vi "斯坦道XML解析.vi"(10 "添加的路径":path, 11 "参数簇":T1={"启动模式"=enum."跨度核查", "启动参数"=1, "量程"=enum."低量程"} {"启动参数" items=["总磷"=1, "总氮"=2, "氨氮"=3]}) -> (2 "步骤时间":string[](array[string]), 3 "步骤名":string[](array[string]))   [LabVIEW 2016, in "斯坦道总氮.lvlib"]
uses:
  <vilib>/xml/Load XML File.vi
  <vilib>/xml/Close Reference(Node).vi
  <resource>/objmgr/DOMUserDefRef.rc
  <vilib>/xml/NI_XML.lvlib
panel:
  out "连接的字符串":string
  out "大小":i32
  out "XML字符串":string="<?xml version=\"1.0\" encoding=\"ISO-8859-1\"?>\n<bookstore>\n<book ISBN=\"978-0545128285\">\n  <title lang=\"en\">The Tales of Beedle the Bard</title>\n  <author>J. K. Rowling</author>\n  <year>2008</year>\n  <price>12.99</price>\n</book>\n<book ISBN=\"978-0316160209\">\n  <title lang=\"en\">Eclipse</title>\n  <author>Stephenie Meyer</author>\n  <year>2007</year>\n  <price>19.99</price>\n</book>\n<book ISBN=\"978-0316067928\">\n  <title lang=\"en\">Breaking Dawn</title>\n  <author>Stephenie Meyer</author>\n  <year>2008</year>\n  <price>22.99</price>\n</book>\n<book ISBN=\"978-0316017923\">\n  <title lang=\"en\">Outliers: The Story of Success</title>\n  <author>Malcolm Gladwell</author>\n  <year>2008</year>\n  <price>27.99</price>\n</book>\n<book ISBN=\"978-0596007645\">\n  <title lang=\"en\">XML in a Nutshell</title>\n  <author>Elliotte Rusty Harold</author>\n  <author>W. Scott Means</author>\n  <year>2004</year>\n  <price>39.95</price>\n</book>\n</bookstore>"
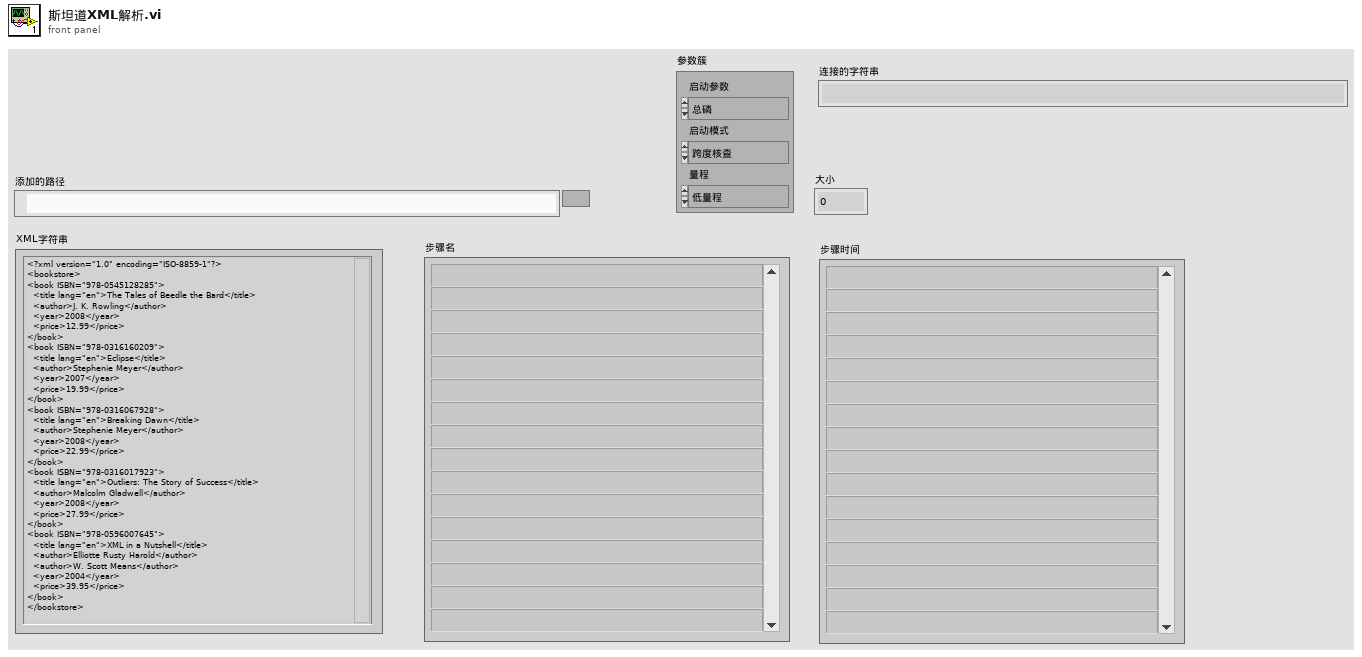
[diagram p1: front panel]
types:
  T1 = cluster{"启动模式":enum16{"跨度核查", "水样测量", "空白核查", "标样核查", "加标回收"}, "启动参数":u16, "量程":enum16{"低量程", "高量程"}}
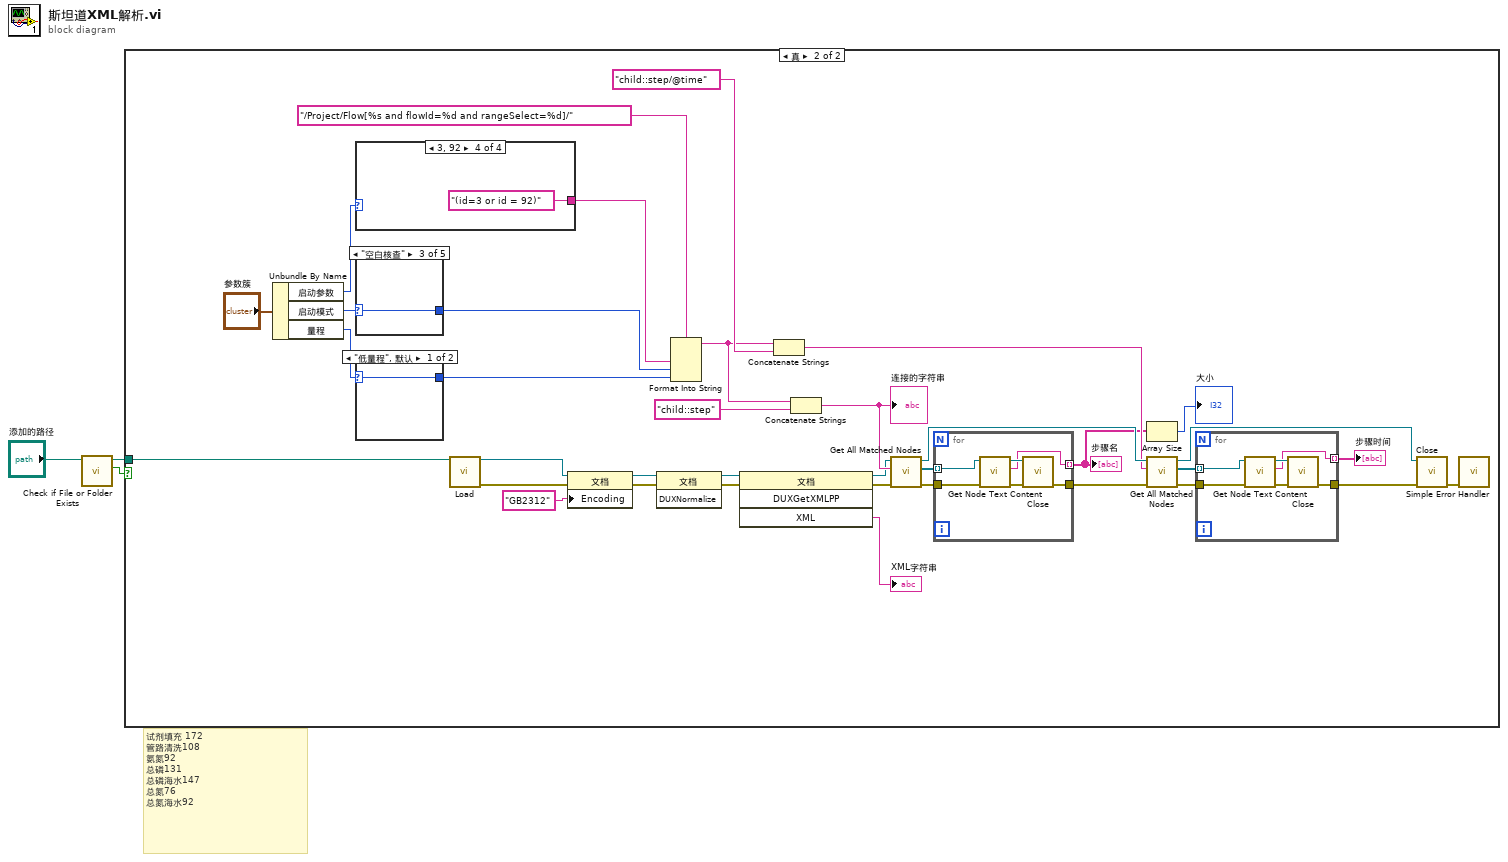
[diagram p0: block diagram]
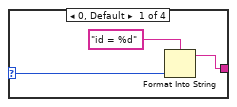
[diagram p3: hidden frame]
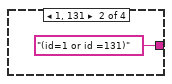
[diagram p4: hidden frame]
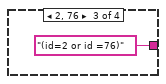
[diagram p5: hidden frame]
diagram:
  # "试剂填充 172 \n管路清洗108\n氨氮92\n总磷131\n总磷海水147\n总氮76\n总氮海水92"
  n1 = call <vilib>:"Check if File or Folder Exists.vi"("path"="添加的路径") -> ("file or folder exists?"=w1:bool, "dup path"=w2:path)  [unwired: 8 in, 1 out]
  n2 = case shown="真" w1 {
    tunnel: w2 -> [_ w4]
    frame False {
    }
    frame True {
      n3 = Unbundle By Name("参数簇") -> ("启动参数"=w6:u16, "启动模式"=w10:enum16{"跨度核查", "水样测量", "空白核查", "标样核查", "加标回收"}, "量程"=w9:enum16{"低量程", "高量程"})
      n4 = case shown="3, 92" w6 {
        selector: w6 -> [w41 _ _ _]
        tunnel: [w40 "(id=1 or id =131)" ("输入 4") "(id=2 or id =76)" ("输入 4") "(id=3 or id = 92)" ("输入 4")] -> w5
        frame 0, Default {
          n5 = Format Into String(format string="id = %d" ("格式字符串"), w41) -> (resulting string=w40:string)  [unwired: 2 in, 1 out]
        }
        frame 1, 131 {
        }
        frame 2, 76 {
        }
        frame 3, 92 {
        }
      }
      n6 = case shown="\"空白核查\"" w10 {
        selector: w10 -> [w54 w55 w56 w57 w58]
        tunnel: [w54 w55 w56 w57 w58] -> w28
        frame "跨度核查", Default {
        }
        frame "水样测量" {
        }
        frame "空白核查" {
        }
        frame "标样核查" {
        }
        frame "加标回收" {
        }
      }
      n7 = case shown="\"低量程\", 默认" w9 {
        selector: w9 -> [w52 w53]
        tunnel: [w52 w53] -> w27
        frame "低量程", Default {
        }
        frame "高量程" {
        }
      }
      n8 = call-poly <vilib>:"Load.vi"("path to XML document"=w4) -> ("DOM document out"=w37:refnum<k20>, "error out"=w36:errorcluster)  [unwired: 12 in, 1 out]
      n9 = property on="属性节点" class="文档"(reference=w37, error in=w36, "Encoding"="GB2312" ("文档编码")) -> (reference out=w35:refnum<k20>, error out=w34:errorcluster)
      n10 = invoke on="Invoke Node" class="文档" method="DUXNormalize"(reference=w35, error in=w34) -> (reference out=w32:refnum<k20>, error out=w33:errorcluster)  [unwired: 1 in, 1 out]
      n11 = Format Into String(format string="/Project/Flow[%s and flowId=%d and rangeSelect=%d]/" ("XPath expression"), w5, w28, w27) -> (resulting string=w16:string)  [unwired: 2 in, 1 out]
      n12 = invoke on="Invoke Node" class="文档" method="DUXGetXMLPP"(reference=w32, error in=w33) -> (reference out=w13:refnum<k20>, error out=w14:errorcluster, "XML"=→"XML字符串":string)  [unwired: 2 in, 1 out]
      n13 = Concatenate Strings(w16, "child::step/@time" ("输入 4")) -> (w17:string)
      n14 = Concatenate Strings(w16, "child::step" ("输入 4")) -> (w19:string)
      "连接的字符串" <- w19
      n15 = call <vilib>:"Get All Matched Nodes.vi"("error in (no error)"=w14, "XPath expression"=w19, "node in"=w13) -> ("error out"=w31:errorcluster, "node result array"=w30:refnum<k20>[], "node out"=w23:refnum<k20>)  [unwired: 6 in]
      n16 = for {
        tunnel: w31 -> [w64]
        tunnel: [w61] -> w8 mode=indexing
        tunnel: w30 -> [w60] mode=indexing
        tunnel: [w59] -> w22
        n17 = call <vilib>:"Get Node Text Content.vi"("error in (no error)"=w64, "node in"=w60) -> ("error out"=w62:errorcluster, "node text"=w61:string, "node out"=w63:refnum<k20>)  [unwired: 7 in]
        n18 = call-poly <vilib>:"Close.vi"("error in (no error)"=w62, "node"=w63) -> ("error out"=w59:errorcluster)  [unwired: 7 out]
      }
      "步骤名" <- w8
      n19 = Array Size(array=w8) -> (size(s)=→"大小":i32)
      n20 = call <vilib>:"Get All Matched Nodes.vi"("error in (no error)"=w22, "XPath expression"=w17, "node in"=w23) -> ("error out"=w25:errorcluster, "node result array"=w24:refnum<k20>[], "node out"=w12:refnum<k20>)  [unwired: 6 in]
      n21 = for {
        tunnel: w25 -> [w51]
        tunnel: [w48] -> w21 mode=indexing
        tunnel: w24 -> [w47] mode=indexing
        tunnel: [w46] -> w15
        n22 = call <vilib>:"Get Node Text Content.vi"("error in (no error)"=w51, "node in"=w47) -> ("error out"=w49:errorcluster, "node text"=w48:string, "node out"=w50:refnum<k20>)  [unwired: 7 in]
        n23 = call-poly <vilib>:"Close.vi"("error in (no error)"=w49, "node"=w50) -> ("error out"=w46:errorcluster)  [unwired: 7 out]
      }
      "步骤时间" <- w21
      n24 = call-poly <vilib>:"Close.vi"("error in (no error)"=w15, "node"=w12) -> ("error out"=w26:errorcluster)  [unwired: 7 out]
      n25 = call <vilib>:"Simple Error Handler.vi"("error in (no error)"=w26) -> ()  [unwired: 4 in, 5 out]
    }
  }
